vi "Read Description.vi"(9 "Control in":refnum<class "Control.lvclass">) -> (3 "Control out":refnum<class "Control.lvclass">, 4 "Description":string)   [LabVIEW 2014, in "Control.lvclass"]
uses:
  Control.lvclass
  Control.lvclass/Control.ctl
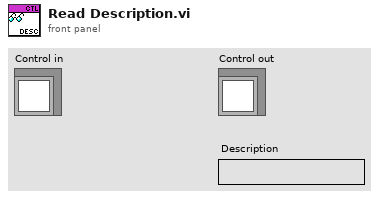
[diagram p1: front panel]
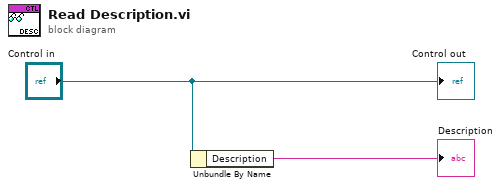
[diagram p0: block diagram]
diagram:
  n1 = Unbundle By Name("Control in") -> ("Description"=→"Description":string)
  "Control out" <- "Control in"
